vi "Read RJDJ Measurement.vi"(0 "VISA resource name":refnum<visa-resource-name>, 5 "Maximum Time (10000ms)":u32=10000, 11 "error in (no error)":errorcluster) -> (1 "BUJ":T2, 2 "Misc":T1, 3 "TJ":T2, 4 "VISA resource name out":refnum<visa-resource-name>, 6 "RJ":T2, 8 "DJ":T2, 10 "PJ":T3, 12 "DDJ":T2, 13 "DCD":cluster{"Result":dbl, "State":i32}, 14 "ISI":T2, 15 "error out":errorcluster)   [LabVIEW 2013, in "Agilent 90000 Series.lvlib"]
doc: "Reads all the RJDJ measurements. It initiates, waits for the acquisition to finish and returns the results of the RJDJ measurement."
uses:
  Agilent 90000 Series.lvlib
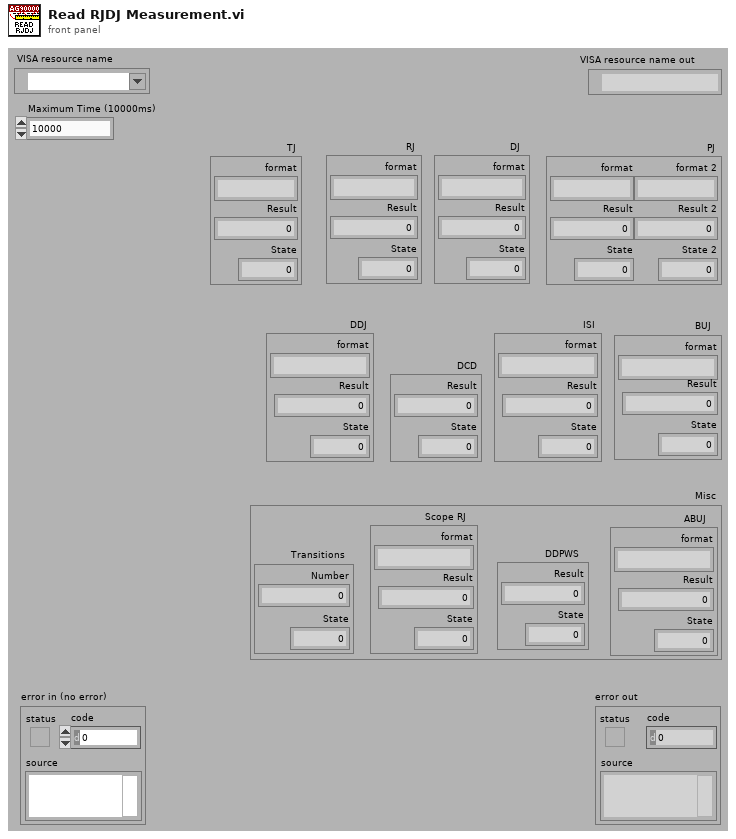
[diagram p1: front panel]
types:
  T1 = cluster{"Transitions":cluster{"Number":dbl, "State":i32}, "Scope RJ":cluster{"format":string, "Result":dbl, "State":i32}, "DDPWS":cluster{"Result":dbl, "State":i32}, "ABUJ":cluster{"format":string, "Result":dbl, "State":i32}}
  T2 = cluster{"format":string, "Result":dbl, "State":i32}
  T3 = cluster{"format":string, "Result":dbl, "State":i32, "format 2":string, "Result 2":dbl, "State 2":i32}
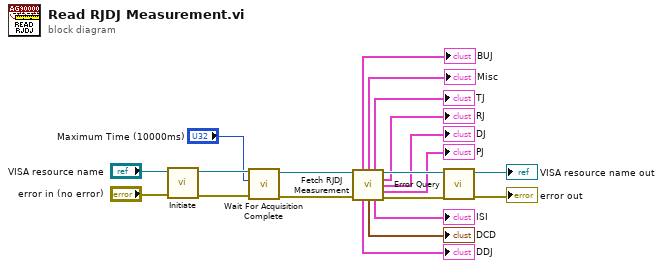
[diagram p0: block diagram]
diagram:
  n1 = call "Initiate.vi"("error in (no error)"="error in (no error)", "VISA resource name"="VISA resource name") -> ("error out"=w17:errorcluster, "VISA resource name out"=w18:refnum<visa-resource-name>)  [unwired: 8 out]
  n2 = call "Wait For Acquisition Complete.vi"("error in (no error)"=w17, "Maximum Time (10000ms)"="Maximum Time (10000ms)", "VISA resource name"=w18) -> ("error out"=w12:errorcluster, "VISA resource name out"=w13:refnum<visa-resource-name>)  [unwired: 7 out]
  n3 = call "Fetch RJDJ Measurement.vi"("VISA resource name"=w13, "error in (no error)"=w12) -> ("BUJ"=→"BUJ":T2, "Misc"=→"Misc":T1, "TJ"=→"TJ":T2, "VISA resource name out"=w11:refnum<visa-resource-name>, "RJ"=→"RJ":T2, "DJ"=→"DJ":T2, "PJ"=→"PJ":T3, "DDJ"=→"DDJ":T2, "DCD"=→"DCD":cluster{"Result":dbl, "State":i32}, "ISI"=→"ISI":T2, "error out"=w10:errorcluster)  [unwired: 3 out]
  n4 = call "Error Query.vi"("error in (no error)"=w10, "VISA resource name"=w11) -> ("error out"=→"error out":errorcluster, "VISA resource name out"=→"VISA resource name out":refnum<visa-resource-name>)  [unwired: 8 out]
